vi "Test_Acquire.vi"() -> ()   [LabVIEW 2019]
uses:
  ClassLoader.lvlib
  <vilib>/Utility/Data Type/Member VI Info.ctl
  Sub/Ctl/Ctl_Class Info.ctl
panel:
  out "Is Interface":bool
  out "Class Info":T1
  out "Hierarchy Array":T1[](array[typedef])
  out "Member VI info":T2[](array[typedef])
  out "error out":errorcluster
  in  "error in":errorcluster
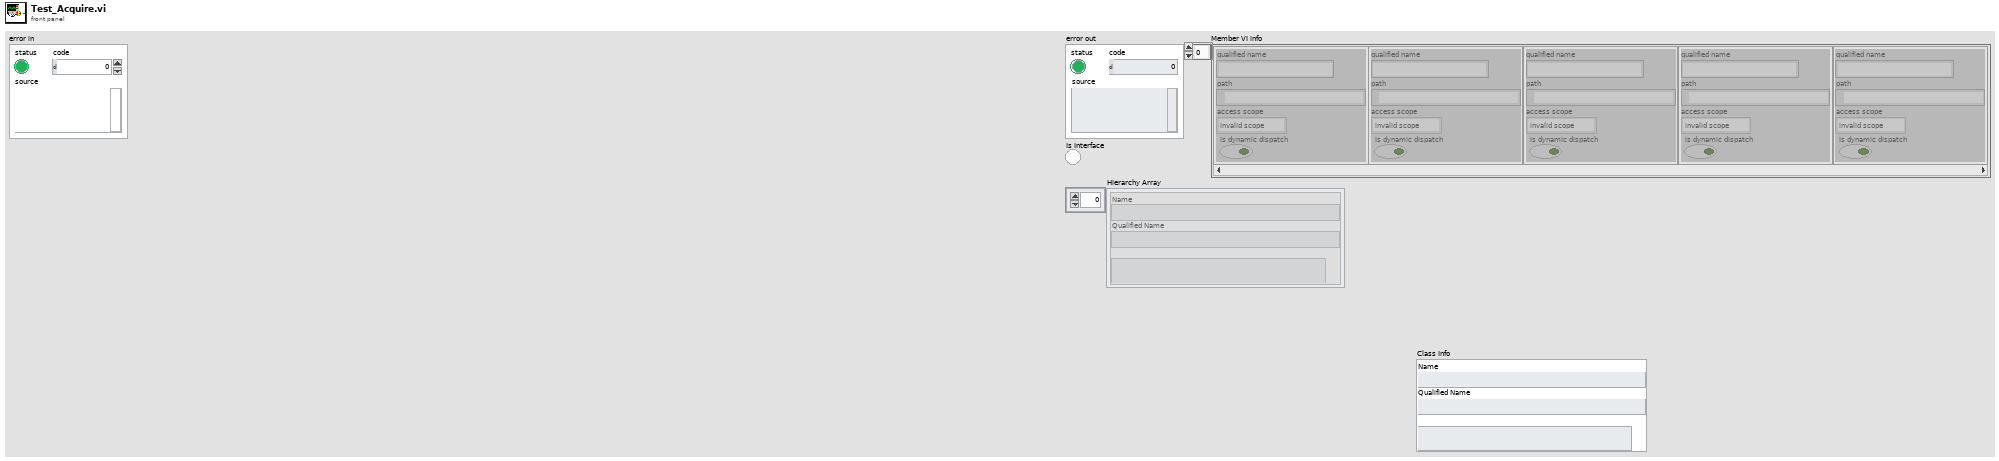
[diagram p1: front panel]
types:
  T1 = typedef "ClassLoader.lvlib/Ctl_Class Info.ctl" = cluster{"Name":string, "Qualified Name":string, "Internal Path":string}
  T2 = typedef "Member VI Info.ctl" = cluster{"qualified name":string, "path":path, "access scope":enum32{"invalid scope", "public", "private", "protected", "community"}, "is dynamic dispatch":bool}
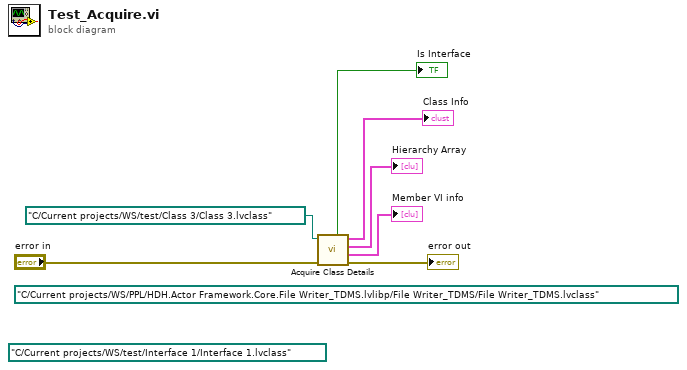
[diagram p0: block diagram]
diagram:
  (unwired) path "C:/Current projects/WS/test/Interface 1/Interface 1.lvclass"
  (unwired) path "C:/Current projects/WS/PPL/HDH.Actor Framework.Core.File Writer_TDMS.lvlibp/File Writer_TDMS/File Writer_TDMS.lvclass" ("Class Path 2")
  n1 = call "Acquire Class Details.vi"("error in"="error in", "Class Path"=path "C:/Current projects/WS/test/Class 3/Class 3.lvclass" ("Class Path 2")) -> ("error out"=→"error out":errorcluster, "Member VI info"=→"Member VI info":T2[], "Hierarchy Array"=→"Hierarchy Array":T1[], "Class Info"=→"Class Info":T1, "Is Interface"=→"Is Interface":bool)  [unwired: 5 in]
